vi "Sim with delay.vi"(6 "T_env":dbl, 8 "theta_d":dbl=1.0, 9 "theta_t":dbl, 10 "Kh":dbl, 11 "u":dbl) -> (3 "T_out":dbl)   [LabVIEW 2019]
uses:
  <vilib>/Simulation/Implementation/Shared/SIMSCR Execution Mode.ctl
  <vilib>/Simulation/Scripting/Companion Diagram/SimConfigNode/SimParams.ctl
  <vilib>/Simulation/Scripting/Companion Diagram/SimConfigNode/_simSolvers.ctl
  <vilib>/Simulation/Param Hierarchy/Typedefs/SIMPH Param Control Actions.ctl
  <vilib>/Simulation/Implementation/Shared/SIM limit type.ctl
  <vilib>/Simulation/Implementation/Shared/NILVSim_ParamChanged.vi
  <vilib>/Simulation/Implementation/Shared/NILVSIM_BeginStep.vi
  <vilib>/Simulation/ContinuousLinear/Implementation/NILVSim Integrator new.llb/SIM Integrator distributor (scalar).vi
  <vilib>/Simulation/ContinuousLinear/Implementation/NILVSim Transport Delay.llb/SIM Transport Delay Distributor (scalar).vi
  <vilib>/Simulation/ContinuousLinear/Implementation/NILVSim Transport Delay.llb/SIM Transport Delay Collector (scalar).vi
  <vilib>/Simulation/ContinuousLinear/Implementation/NILVSim Integrator new.llb/SIM Integrator collector (scalar).vi
  <vilib>/Simulation/Implementation/Shared/NILVSim_Manager.vi
  <vilib>/Utility/error.llb/Clear Errors.vi
  <vilib>/Simulation/Implementation/Shared/NILVSim_FinalizeModel.vi
  <vilib>/Simulation/Implementation/Shared/SIM Unbundle Sim Info.vi
  <vilib>/Simulation/Implementation/Shared/SIMSH Read Queue.vi
  <vilib>/Simulation/Implementation/Shared/NILVSim_Initialize.vi
  <vilib>/Simulation/Utility/Implementation/NILVSim Get Time and IsAcceptedStep.vi
  <vilib>/Simulation/Implementation/Shared/NILVSim_GetModelError.vi
  <vilib>/Simulation/Implementation/Shared/SIM SimErrorHandler.vi
  <vilib>/Simulation/Implementation/Shared/SIM Bundle Sim Info.vi
  <vilib>/Simulation/Scripting/Companion Diagram/SimConfigNode/SimDog.xnode
  <vilib>/Simulation/Implementation/XNodeFramework/SimXNode/SimX.xnode
  <vilib>/Simulation/ContinuousLinear/Implementation/NILVSim Integrator new.llb/SIM Integrator (scalar).vi
  <vilib>/Simulation/ContinuousLinear/Implementation/NILVSim Transport Delay.llb/SIM Transport Delay Indirect (scalar).vi
  <vilib>/Simulation/Implementation/Shared/NI_SIM_Implementation.lvlib
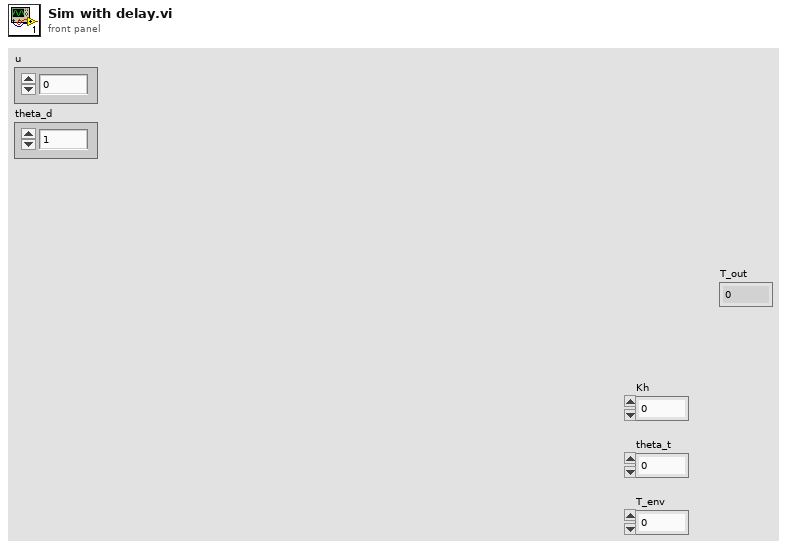
[diagram p1: front panel]
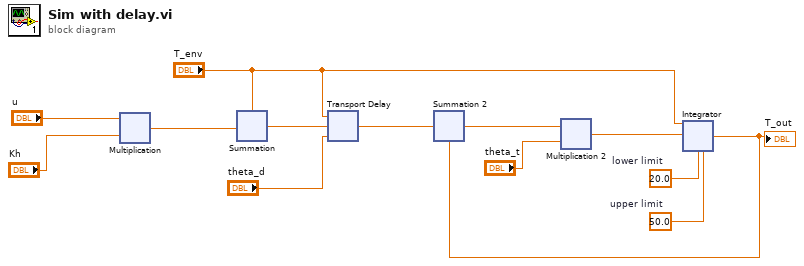
[diagram p0: block diagram]
diagram:
  w3 = 50.0  # upper limit
  w4 = 20.0  # lower limit
  n1 = xnode "Multiplication"("Operand1"="u", "Operand2"="Kh") -> ("Result"=w11:dbl)
  n2 = xnode "Summation"("Operand1"="T_env", "Operand2"=w11) -> ("Result"=w10:dbl)
  n3 = xnode "Transport Delay"("initial condition"="T_env", "input"=w10, "delay (s)"="theta_d") -> ("output"=w8:dbl)  [unwired: 2 in]
  n4 = xnode "Summation 2"("Operand1"=w8, "Operand2"=w2) -> ("Result"=w7:dbl)
  n5 = xnode "Multiplication 2"("Operand1"=w7, "Operand2"="theta_t") -> ("Result"=w6:dbl)
  n6 = xnode "Integrator"("upper limit"=w3, "input"=w6, "initial condition"="T_env", "lower limit"=w4) -> ("output"=w2:dbl)  [unwired: 6 in, 2 out]
  "T_out" <- w2
